vi "Initialize.vi"(8 "错误输入（无错误）":errorcluster, 11 "Super Data Model in":refnum<class "Super Data Model.lvclass">) -> (0 "错误输出":errorcluster, 3 "Super Data Model out":refnum<class "Super Data Model.lvclass">)   [LabVIEW 2013, in "Modbus Library - Advance.lvlib" / "Super Data Model.lvclass"]
uses:
  Super Data Model.lvclass
  Standard Data Model/Standard Data Model.lvclass
  Super Data Model.lvclass/Super Data Model.ctl
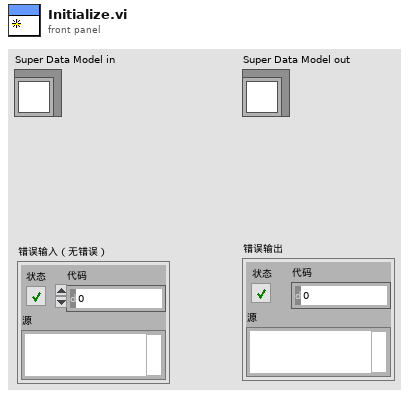
[diagram p1: front panel]
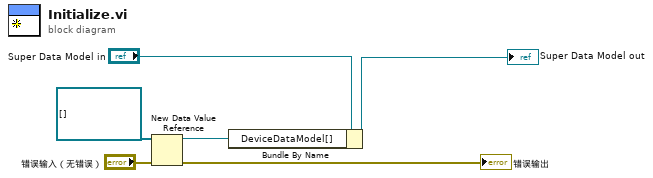
[diagram p0: block diagram]
diagram:
  n1 = New Data Value Reference(data value=refnum<class "Standard Data Model.lvclass">[] [], error in="错误输入（无错误）") -> (data value reference=w3:refnum<data-value>, error out=→"错误输出":errorcluster)
  n2 = Bundle By Name(cluster="Super Data Model in", "DeviceDataModel[]"=w3) -> (→"Super Data Model out":refnum<class "Super Data Model.lvclass">)
